vi "Init Digitizers.vi"(6 "NI Cards":i32=3, 8 "Bypass 2nd Digitizer Init":bool, 9 "Digitizer Config":i32(ring)=4 items=["Single channel"=0, "2 Chans w/ 2 Acqiris"=1, "2 Chans w/ 1 Acqiris"=2, "5-CH pulser w/ ann array"=4, "5-pass style ann array"=5], 10 "Main Digitizer":T2=enum."NI Digitizer", 11 "Digitizer Settings in":T1={"Digitizer delay (us) "=0.0, "rf points per line"=0, "lines per plane"=0, "Samp Rate (Hz)"=0.0, "Additional dig delay (us)"=0.0, "Voltage Scale"=0.0, "Pre-Looks"=0, "Offset delay (us)"=0.0, "bits A/D"=0, "Avg Num"=0, "DigTimeOut"=0.0, "Rel Dig Delay"=0.0, "Dig Ch"=0, "LeCroyCluster"={"LeCroy Channels"=[], "LC read pt offset"=0.0, "Sweep Avg"=FALSE}, "Main Digitizer"=enum."Acqiris Digitizer", "Dig Config"=enum."Single channel", "Digitizer ID Cluster"={"Acqiris/Alazar/SP ID"=[], "NI Instr Handles"=[], "LeCroy VISA"="", "GaGe Handle"={"Handle"=0, "Sample size"=0, "Resolution"=0, "Offset"=0, "Channels"=0, "Boards"=0}, "ATS Ref"="", "Acqiris Address"=[], "ADQRef"=refnum, "adq_cu_ptr"=refnum}, "Trigger Settings"={"Trig Source"=0, "Trig Coupling"=0, "Trig Slope"=0, "Level (mV)"=0.0}, "Bulk Acq"=FALSE, "Bulk Start Indexes"=[], "Data Ref RF"=refnum, "NI ID/Channel"=[], "Total Dig CH"=5, "Xtra Ann Trig delay (us)"=10.0, "Fix Z Delay?"=FALSE, "One Way Transmission?"=FALSE, "Data Ref Log"=refnum} {"Trigger Settings"."Trig Slope" items=["Positive", "Negative"]; "Trigger Settings"."Level (mV)" format="%.2f"; "Trigger Settings"."Trig Coupling" items=["DC 1 MOhm", "AC 1 MOhm", "DC 50 Ohm", "AC 50 Ohm"]; "Trigger Settings"."Trig Source" items=["Chan 1", "External"]; "Rel Dig Delay" format="%.2f"; "DigTimeOut" format="%.2f"; "Avg Num" min=1; "Offset delay (us)" format="%.2f"; "Additional dig delay (us)" format="%.2f"; "Digitizer delay (us)" format="%.2f"}) -> (0 "Bypass 2nd Digitizer Init":bool, 1 "Initialization Failed!!":bool, 3 "Digitizer Settings":T1={"Digitizer delay (us) "=0.0, "rf points per line"=0, "lines per plane"=0, "Samp Rate (Hz)"=0.0, "Additional dig delay (us)"=0.0, "Voltage Scale"=0.0, "Pre-Looks"=0, "Offset delay (us)"=0.0, "bits A/D"=0, "Avg Num"=0, "DigTimeOut"=0.0, "Rel Dig Delay"=0.0, "Dig Ch"=0, "LeCroyCluster"={"LeCroy Channels"=[], "LC read pt offset"=0.0, "Sweep Avg"=FALSE}, "Main Digitizer"=enum."Acqiris Digitizer", "Dig Config"=enum."Single channel", "Digitizer ID Cluster"={"Acqiris/Alazar/SP ID"=[], "NI Instr Handles"=[], "LeCroy VISA"="", "GaGe Handle"={"Handle"=0, "Sample size"=0, "Resolution"=0, "Offset"=0, "Channels"=0, "Boards"=0}, "ATS Ref"="", "Acqiris Address"=[], "ADQRef"=refnum, "adq_cu_ptr"=refnum}, "Trigger Settings"={"Trig Source"=0, "Trig Coupling"=0, "Trig Slope"=0, "Level (mV)"=0.0}, "Bulk Acq"=FALSE, "Bulk Start Indexes"=[], "Data Ref RF"=refnum, "NI ID/Channel"=[], "Total Dig CH"=5, "Xtra Ann Trig delay (us)"=10.0, "Fix Z Delay?"=FALSE, "One Way Transmission?"=FALSE, "Data Ref Log"=refnum} {"Trigger Settings"."Trig Slope" items=["Positive", "Negative"]; "Trigger Settings"."Level (mV)" format="%.2f"; "Trigger Settings"."Trig Coupling" items=["DC 1 MOhm", "AC 1 MOhm", "DC 50 Ohm", "AC 50 Ohm"]; "Trigger Settings"."Trig Source" items=["Chan 1", "External"]; "Rel Dig Delay" format="%.2f"; "DigTimeOut" format="%.2f"; "Avg Num" min=1; "Offset delay (us)" format="%.2f"; "Additional dig delay (us)" format="%.2f"; "Digitizer delay (us)" format="%.2f"})   [LabVIEW 2022 SP3]
uses:
  <instrlib>/Acqiris Dx/Acqiris Dx.lvlib
  <instrlib>/Acqiris Bx/Acqiris Bx.lvlib
  <instrlib>/niScope/Controls/niScope input clock source.ctl
  <instrlib>/LeCroy Wave Series/LeCroy Wave Series.lvlib
  C:/AlazarTech/ATS-VI/6.2.0/ATS_ctl/Device_Ctrl.ctl
  C:/AlazarTech/ATS-VI/6.2.0/ATS_ctl/ATS_Check_Ctrl.ctl
  Digitizer.ctl
  DigitizerID.ctl
  DigitizerSettings.ctl
  DigConfig.ctl
  C:/Windows/System32/ADQAPI_dotNet_helper.dll
panel:
  out "error out":errorcluster
  in  "error in (no error)":errorcluster
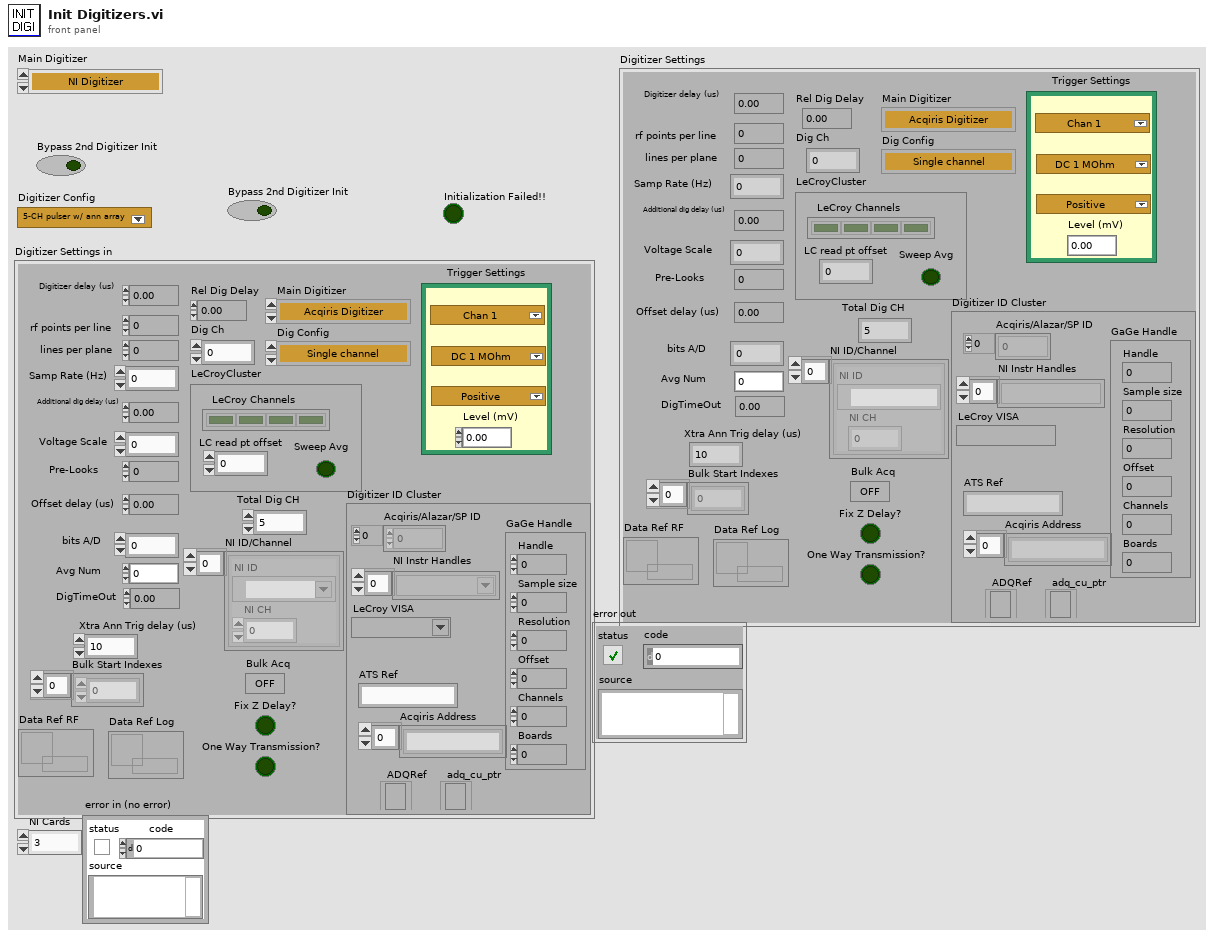
[diagram p1: front panel]
types:
  T1 = typedef "DigitizerSettings.ctl" = cluster{"Digitizer delay (us) ":dbl, "rf points per line":i32, "lines per plane":i32, "Samp Rate (Hz)":dbl, "Additional dig delay (us)":dbl, "Voltage Scale":dbl, "Pre-Looks":i32, "Offset delay (us)":dbl, "bits A/D":i8, "Avg Num":i32, "DigTimeOut":sgl, "Rel Dig Delay":sgl, "Dig Ch":i32, "LeCroyCluster":cluster{"LeCroy Channels":bool[], "LC read pt offset":dbl, "Sweep Avg":bool}, "Main Digitizer":T2, "Dig Config":T3, "Digitizer ID Cluster":T4, "Trigger Settings":cluster{"Trig Source":u16, "Trig Coupling":u16, "Trig Slope":u16, "Level (mV)":dbl}, "Bulk Acq":bool, "Bulk Start Indexes":i32[], "Data Ref RF":refnum<data-value>, "NI ID/Channel":cluster{"NI ID":refnum<k15>, "NI CH":i32}[], "Total Dig CH":i32, "Xtra Ann Trig delay (us)":dbl, "Fix Z Delay?":bool, "One Way Transmission?":bool, "Data Ref Log":refnum<data-value>}
  T2 = typedef "Digitizer.ctl" = enum16{"Acqiris Digitizer", "NI Digitizer", "LeCroy", "GaGe", "AlazarTech", "No Digitizer", "Teledyne"}
  T3 = typedef "DigConfig.ctl" = enum16{"Single channel", "2 Chans w/ 2 Acqiris", "2 Chans w/ 1 Acqiris", "5-CH Pulser New", "5-CH pulser w/ ann array", "5-pass style ann array", "Empty"}
  T4 = typedef "DigitizerID.ctl" = cluster{"Acqiris/Alazar/SP ID":u32[], "NI Instr Handles":refnum<k15>[], "LeCroy VISA":refnum<visa-resource-name>, "GaGe Handle":cluster{"Handle":u32, "Sample size":u32, "Resolution":i32, "Offset":i32, "Channels":u32, "Boards":u32}, "ATS Ref":string, "Acqiris Address":string[], "ADQRef":refnum<k24>, "adq_cu_ptr":refnum<k24>}
  T5 = typedef "ATS_Check_Ctrl.ctl" = enum16{"None", "NO_ATS9462", "ATS9462_Traditional", "Verify Board", "OnBoard Memory", "Board & Memory", "Master/Slave", "NO Master/Slave"}
  T6 = typedef "Device_Ctrl.ctl" = enum16{"Status", "About", "Arm", "ForceTrig", "Abort", "Initialize", "Init (NoPreset)", "Info", "Close", "Calibrate", "SetManually", "LED_ON", "LED_OFF"}
  T7 = typedef "niScope input clock source.ctl" = u16
  T8 = cluster{"Handle":u32, "Sample size":u32, "Resolution":i32, "Offset":i32, "Channels":u32, "Boards":u32}
  T9 = typedef "Device_Info.ctl" = cluster{"Handle":u32, "Board":string, "CPLD":string, "MemorySize":u32, "SampleSize":u8, "ID":i32, "High_Memory":bool, "Chan/Board":u8}
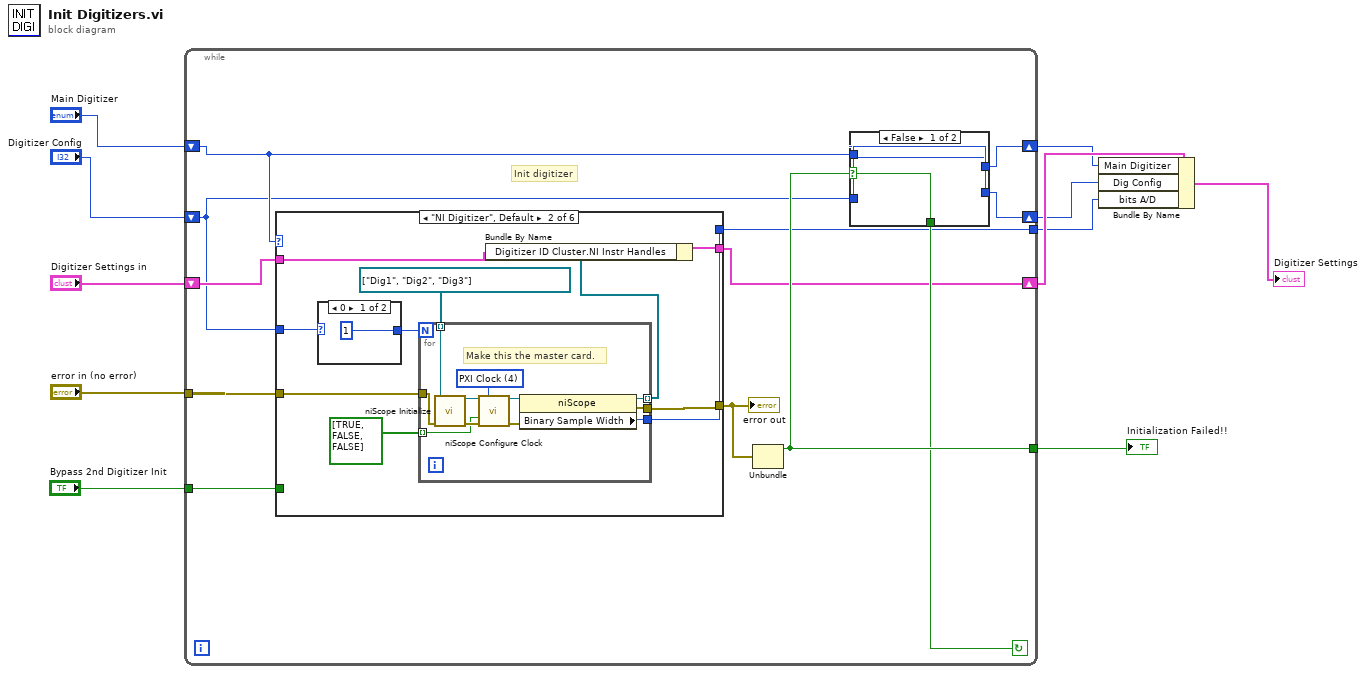
[diagram p0: block diagram]
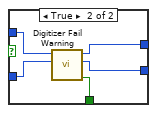
[diagram p2: hidden frame]
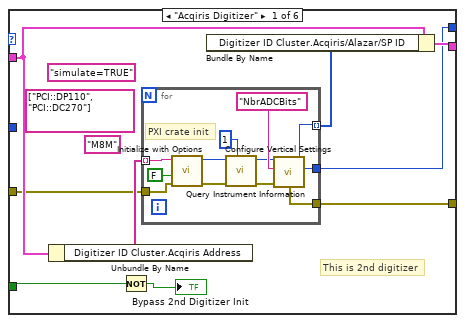
[diagram p3: hidden frame]
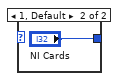
[diagram p4: hidden frame]
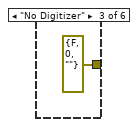
[diagram p5: hidden frame]
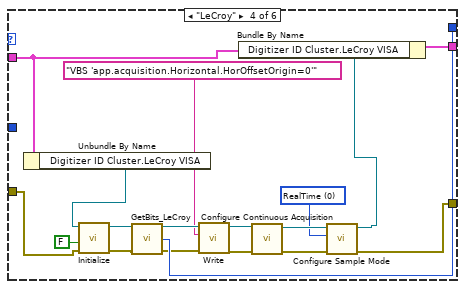
[diagram p6: hidden frame]
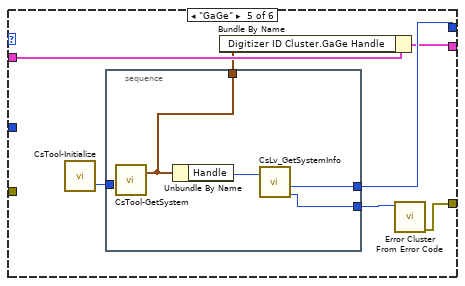
[diagram p7: hidden frame]
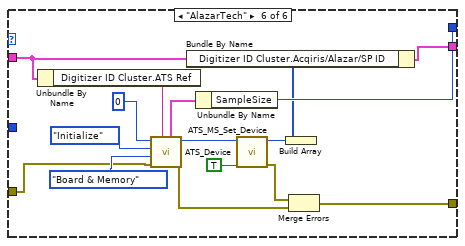
[diagram p8: hidden frame]
diagram:
  n1 = while {
    tunnel: "Bypass 2nd Digitizer Init" -> [w23]
    tunnel: "error in (no error)" -> [w21]
    tunnel: [w19] -> w8
    shift-right: [w12] -> w5
    shift-left: "Digitizer Settings in" -> [w22]
    shift-right: [w17] -> w2
    shift-left: "Digitizer Config" -> [w14]
    shift-right: [w16] -> w3
    shift-left: "Main Digitizer" -> [w15]
    tunnel: [w13] -> w1
    stop <- w18 continue-if-true
    # "Init digitizer"
    n2 = case shown="\"NI Digitizer\", Default" w15 {
      tunnel: [w37 w62 _ w91 w101 w115] -> w13
      tunnel: w23 -> [w40 _ _ _ _ _]
      tunnel: w14 -> [_ w59 _ _ _ _]
      tunnel: w22 -> [w36 w57 _ w80 w99 w110]
      tunnel: [w39 w56 _ w81 w97 w112] -> w12
      tunnel: [w33 w54 errorcluster {"status"=FALSE, "code"=0, "source"=""} ("error IO") w78 w95 w107] -> w20
      tunnel: w21 -> [w32 w53 _ w77 _ w109]
      frame "Acqiris Digitizer" {
        (unwired) "M8M" ("Options String (null string)")
        (unwired) string[] ["PCI::DP110", "PCI::DC270"]
        (unwired) "simulate=TRUE" ("Options String (null string)")
        # "This is 2nd digitizer"
        n3 = Unbundle By Name(w36) -> ("Digitizer ID Cluster.Acqiris Address"=w35:string[])
        n4 = Not(x=w40) -> (.not. x?=→"Bypass 2nd Digitizer Init":bool)
        n5 = for {
          tunnel: [w45] -> w38 mode=indexing
          tunnel: w35 -> [w48] mode=indexing
          tunnel: [w43] -> w37
          tunnel: [w42] -> w33
          tunnel: w32 -> [w41]
          # "PXI crate init"
          n6 = call <instrlib>:"Initialize with Options.vi"("Resource Name (PCI::INSTR0)"=w48, "Reset (T: Reset)"=FALSE, "error in (no error)"=w41) -> ("Instrument ID"=w51:u32, "error out"=w50:errorcluster)  [unwired: 3 in, 2 out]
          n7 = call <instrlib>:"Configure Vertical Settings.vi"("Channel (1)"=1, "error in (no error)"=w50, "Instrument ID"=w51) -> ("error out"=w44:errorcluster, "dup Instrument ID"=w46:u32)  [unwired: 4 in, 3 out]
          n8 = call <instrlib>:"Query Instrument Information.vi"("Instrument ID"=w46, "Parameter String"="NbrADCBits", "error in (no error)"=w44) -> ("dup Instrument ID"=w45:u32, "Info Value (I32)"=w43:i32, "error out"=w42:errorcluster)  [unwired: 1 in, 3 out]
        }
        n9 = Bundle By Name(cluster=w36, "Digitizer ID Cluster.Acqiris/Alazar/SP ID"=w38) -> (w39:T1)
      }
      frame "NI Digitizer", Default {
        n10 = case shown="0" w59 {
          tunnel: [1 "NI Cards"] -> w58
          frame 0 {
          }
          frame 1, Default {
          }
        }
        n11 = for {
          N: w58 -> [_]
          tunnel: [w71] -> w55 mode=indexing
          tunnel: [w69] -> w62
          tunnel: refnum<k15>[] ["Dig1", "Dig2", "Dig3"] -> [w68] mode=indexing
          tunnel: bool[] [TRUE, FALSE, FALSE] -> [w67] mode=indexing
          tunnel: [w66] -> w54
          tunnel: w53 -> [w65]
          w73 = T7 4 items=["None"=0, "RTSI Clock"=1, "PFI 0"=6, "PFI 1"=2, "PFI 2"=3, "PXI Clock"=4, "External"=5, "Clock In"=7] ("input clock source")
          # "Make this the master card."
          n12 = call <instrlib>:"niScope Initialize.vi"("resource name"=w68, "error in"=w65) -> ("instrument handle"=w75:refnum<k15>, "error out"=w74:errorcluster)  [unwired: 2 in, 10 out]
          n13 = call <instrlib>:"niScope Configure Clock.vi"("instrument handle"=w75, "input clock source"=w73, "master enabled"=w67, "error in"=w74) -> ("instrument handle out"=w72:refnum<k15>, "error out"=w70:errorcluster)  [unwired: 2 in, 8 out]
          n14 = property class="niScope"(reference=w72, error in=w70) -> (reference out=w71:refnum<k15>, error out=w66:errorcluster, "Binary Sample Width"=w69:i32)
        }
        n15 = Bundle By Name(cluster=w57, "Digitizer ID Cluster.NI Instr Handles"=w55) -> (w56:T1)
      }
      frame "No Digitizer" {
      }
      frame "LeCroy" {
        w88 = u16 0 items=["RealTime", "RIS", "Sequence", "Roll", "WaveStream"] ("Sample Mode (0: RealTime)")
        n16 = Unbundle By Name(w80) -> ("Digitizer ID Cluster.LeCroy VISA"=w79:refnum<visa-resource-name>)
        n17 = call <instrlib>:"Initialize.vi"("error in (no error)"=w77, "Reset? (T: Yes)"=FALSE, "VISA resource name"=w79) -> ("error out"=w92:errorcluster, "VISA resource name out"=w93:refnum<visa-resource-name>)  [unwired: 7 in]
        n18 = call "GetBits_LeCroy.vi"("VISA resource name"=w93, "error in (no error)"=w92) -> ("VISA resource name out"=w84:refnum<visa-resource-name>, "Nom_Bits"=w91:i16, "error out"=w85:errorcluster)  [unwired: 11 in]
        n19 = call <instrlib>:"Write.vi"("error in (no error)"=w85, "Write Buffer"="VBS 'app.acquisition.Horizontal.HorOffsetOrigin=0'", "VISA resource name"=w84) -> ("error out"=w86:errorcluster, "VISA resource name out"=w87:refnum<visa-resource-name>)  [unwired: 6 in, 1 out]
        n20 = call <instrlib>:"Configure Continuous Acquisition.vi"("error in (no error)"=w86, "VISA resource name"=w87) -> ("error out"=w90:errorcluster, "VISA resource name out"=w89:refnum<visa-resource-name>)  [unwired: 8 in]
        n21 = call <instrlib>:"Configure Sample Mode.vi"("error in (no error)"=w90, "Sample Mode (0: RealTime)"=w88, "VISA resource name"=w89) -> ("error out"=w78:errorcluster, "VISA resource name out"=w82:refnum<visa-resource-name>)  [unwired: 7 in]
        n22 = Bundle By Name(cluster=w80, "Digitizer ID Cluster.LeCroy VISA"=w82) -> (w81:T1)
      }
      frame "GaGe" {
        n23 = call <userlib>:"CsTool-Initialize.vi"() -> ("Error Code"=w100:i32)  [unwired: 1 out]
        n24 = stacked-sequence {
          tunnel: [w104] -> w101
          tunnel: w100 -> [_]
          tunnel: [w103] -> w98
          tunnel: [w102] -> w96
          frame #0 {
            n25 = call <userlib>:"CsTool-GetSystem.vi"() -> ("Handle Cluster"=w103:T8)  [unwired: 4 in, 1 out]
            n26 = Unbundle By Name(w103) -> ("Handle"=w105:u32)
            n27 = call <userlib>:"CsLv_GetSystemInfo.vi"("Handle"=w105) -> ("Sample Bits"=w104:u32, "Error Code"=w102:i32)  [unwired: 5 out]
          }
        }
        n28 = Bundle By Name(cluster=w99, "Digitizer ID Cluster.GaGe Handle"=w98) -> (w97:T1)
        n29 = call <vilib>:"Error Cluster From Error Code.vi"("error code (0)"=w96) -> ("error out"=w95:errorcluster)  [unwired: 8 in]
      }
      frame "AlazarTech" {
        n30 = Unbundle By Name(w110) -> ("Digitizer ID Cluster.ATS Ref"=w111:string)
        n31 = call "ATS_Device.vi"("BoardToVerify"=w111, "error in (no error)"=w109, "ATS_Check"=ATS_Check_Ctrl."Board & Memory", "DevCtrl"=Device_Ctrl."Initialize", "DeviceIn"=0) -> ("error out"=w106:errorcluster, "DeviceOut"=w118:i32, "DevInfo"=w116:T9)  [unwired: 4 out]
        n32 = Unbundle By Name(w116) -> ("SampleSize"=w115:u8)
        n33 = call "ATS_MS_Set_Device.vi"("Update_Only"=TRUE, "DeviceIn"=w118) -> ("error out"=w108:errorcluster, "DeviceOut"=w113:i32)  [unwired: 4 in, 4 out]
        n34 = Build Array(w113) -> (w114:i32[])
        n35 = Bundle By Name(cluster=w110, "Digitizer ID Cluster.Acqiris/Alazar/SP ID"=w114) -> (w112:T1)
        n36 = Merge Errors(w108, w106) -> (w107:errorcluster)
      }
    }
    "error out" <- w20
    n37 = Unbundle(w20) -> ("status"=w19:bool)  [unwired: 2 out]
    n38 = case shown="False" w19 {
      selector: w19 -> [w26 _]
      tunnel: w14 -> [w25 w31]
      tunnel: w15 -> [w24 w30]
      tunnel: [w26 w29] -> w18
      tunnel: [w25 w28] -> w17
      tunnel: [w24 w27] -> w16
      frame False {
      }
      frame True {
        n39 = call "Digitizer Fail Warning.vi"("Digitizer Config"=w31, "Main Digitizer"=w30) -> ("Retry"=w29:bool, "Digitizer Config"=w28:i32, "Main Digitizer"=w27:T2)  [unwired: 5 in, 2 out]
      }
    }
  }
  "Initialization Failed!!" <- w8
  n40 = Bundle By Name(cluster=w5, "Main Digitizer"=w3, "Dig Config"=w2, "bits A/D"=w1) -> (→"Digitizer Settings":T1)
